vi "_Parse Markdown Note Elements.vi"(8 "Error in":errorcluster caption="Error in (no error)", 11 "Lines":string[](array[string])) -> (0 "Error out":errorcluster, 2 "Array":T1[](array[typedef]), 3 "Lines (dup)":string[](array[string]))   [LabVIEW 2017, in "csmdoc.lvlib"]
uses:
  csmdoc.lvlib
  _Typedef/DocNote.ctl
  _tool/_file/csm-file-support.lvlib
  Communicable State Machine.lvlib
  _Shared/CSM Shared.lvlib
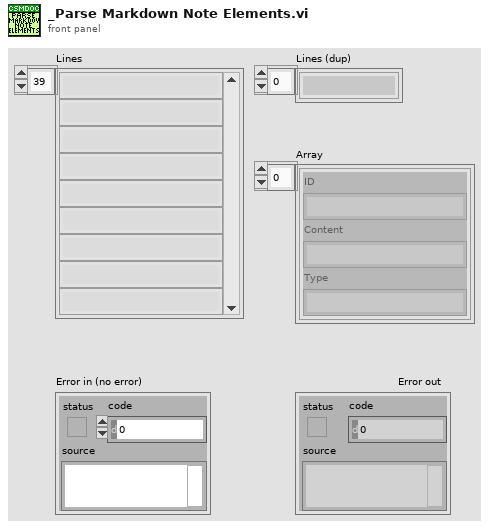
[diagram p1: front panel]
types:
  T1 = typedef "csmdoc.lvlib/DocNote.ctl" = cluster{"ID":string, "Content":string, "Type":string}
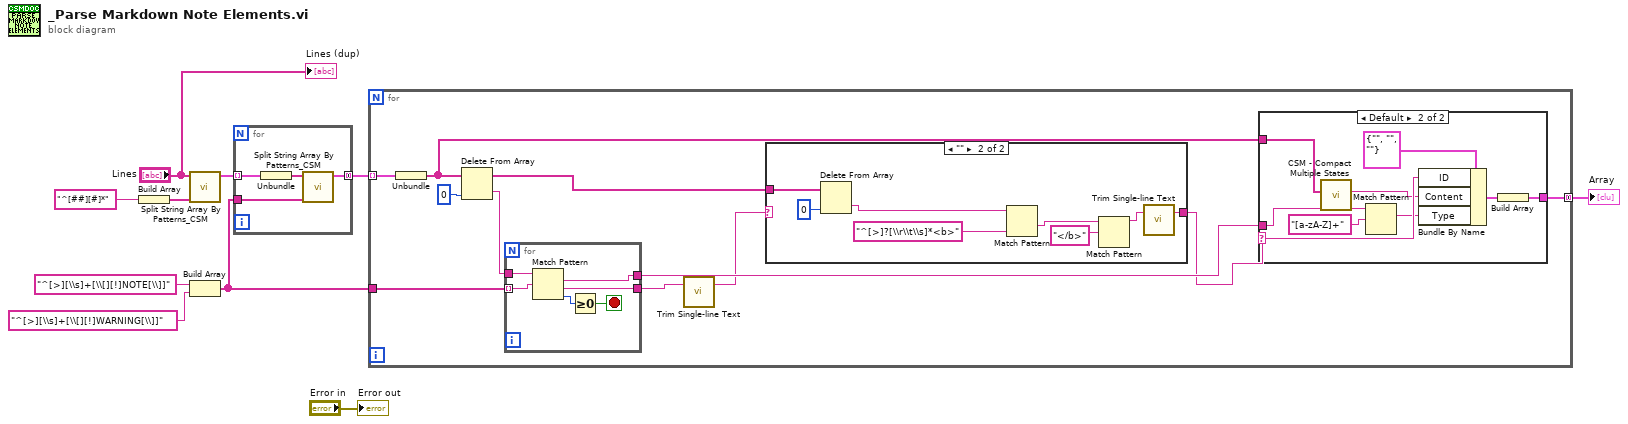
[diagram p0: block diagram]
diagram:
  n1 = Build Array("^[##][#]*" ("delimited string")) -> (w4:string[])
  n2 = call "Split String Array By Patterns_CSM.vi"("Patterns"=w4, "Text Array"="Lines") -> ("Array"=w5:cluster{"filtered array":string[]}[])  [unwired: 9 in]
  n3 = Build Array("^[>][\\s]+[\\[][!]NOTE[\\]]" ("delimited string"), "^[>][\\s]+[\\[][!]WARNING[\\]]" ("delimited string")) -> (w9:string[])
  n4 = for {
    tunnel: w5 -> [w14] mode=indexing
    tunnel: [w12] -> w6 mode=concatenating
    tunnel: w9 -> [w11]
    n5 = Unbundle(w14) -> ("filtered array"=w13:string[])
    n6 = call "Split String Array By Patterns_CSM.vi"("Patterns"=w11, "Text Array"=w13) -> ("Array"=w12:cluster{"filtered array":string[]}[])  [unwired: 9 in]
  }
  n7 = for {
    tunnel: w6 -> [w25] mode=indexing
    tunnel: [w21] -> w10 mode=concatenating
    tunnel: w9 -> [w20]
    n8 = Unbundle(w25) -> ("filtered array"=w18:string[])
    n9 = Delete From Array(array=w18, index=0) -> (deleted portion=w22:string, array with subset deleted=w17:string[])  [unwired: 1 in]
    n10 = for {
      tunnel: w22 -> [w39]
      tunnel: [w40] -> w23
      tunnel: w20 -> [w38] mode=indexing
      tunnel: [w35] -> w19
      stop <- w36 stop-if-true
      n11 = Match Pattern(string=w39, regular expression=w38) -> (match substring=w35:string, after substring=w40:string, offset past match=w37:i32)  [unwired: 1 in, 1 out]
      n12 = Greater Or Equal To 0?(x=w37) -> (x >= 0?=w36:bool)
    }
    n13 = call "Trim Single-line Text.vi"("single-line text"=w23) -> ("trimed text"=w16:string)  [unwired: 2 in]
    n14 = case shown="\"\"" w16 {
      selector: w16 -> [w26 _]
      tunnel: w17 -> [_ w33]
      tunnel: [w26 w27] -> w15
      frame "False", Default {
      }
      frame "" {
        n15 = Delete From Array(array=w33, index=0) -> (deleted portion=w32:string)  [unwired: 1 in, 1 out]
        n16 = Match Pattern(string=w32, regular expression="^[>]?[\\r\\t\\s]*<b>") -> (after substring=w29:string)  [unwired: 1 in, 3 out]
        n17 = Match Pattern(string=w29, regular expression="</b>") -> (before substring=w28:string)  [unwired: 1 in, 3 out]
        n18 = call "Trim Single-line Text.vi"("single-line text"=w28) -> ("trimed text"=w27:string)  [unwired: 2 in]
      }
    }
    n19 = case shown="Default" w15 {
      selector: w15 -> [_ w48]
      tunnel: [_ w45] -> w21
      tunnel: w19 -> [_ w43]
      tunnel: w18 -> [_ w41]
      frame "" {
      }
      frame Default {
        n20 = call "CSM - Compact Multiple States.vi"("Multiple States"=w41) -> ("States"=w47:string)  [unwired: 9 in]
        n21 = Match Pattern(string=w43, regular expression="[a-zA-Z]+") -> (match substring=w42:string)  [unwired: 1 in, 3 out]
        n22 = Bundle By Name(cluster=T1 {"ID"="", "Content"="", "Type"=""} ("Cluster"), "ID"=w48, "Content"=w47, "Type"=w42) -> (w46:T1)
        n23 = Build Array(w46) -> (w45:T1[])
      }
    }
  }
  "Array" <- w10
  "Error out" <- "Error in"
  "Lines (dup)" <- "Lines"
